vi "相机1初始化.vi"() -> (1 "Session Out":T2, 2 "Image":T1, 3 "相机1状态":bool, 4 "error out":errorcluster)   [LabVIEW 2014]
uses:
  <vilib>/userdefined/High Color/IMAQdx.ctl
  <vilib>/vision/Image Controls.llb/IMAQ Image.ctl
  Controls/MsgAction.ctl
  Global.vi
  <vilib>/vision/driver/NI_Vision_Acquisition_Software.lvlib
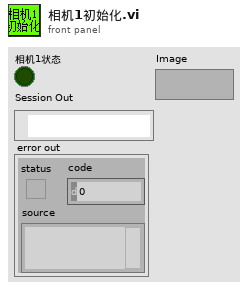
[diagram p1: front panel]
types:
  T1 = typedef "IMAQ Image.ctl" = refnum<image>
  T2 = typedef "IMAQdx.ctl" = refnum<k21>
  T3 = typedef "MsgAction.ctl" = enum16{"初始化", "添加消息", "区分结果添加消息", "清空消息", "获取消息"}
  T4 = typedef "OtherSpec.ctl" = cluster{"其它勾选类规格":T5, "其它数据类规格":T6, "相机名称":T7, "参数":cluster{"Mark1曝光时间":i32, "Mark2曝光时间":i32, "二维码曝光时间":i32}}
  T5 = typedef "其它勾选类规格.ctl" = cluster{"保存图片":bool, "上传设备状态数据":bool, "保存数据":bool, "开机默认开启监控摄像头":bool, "启用mark拍照 ":bool}
  T6 = typedef "其他数据类规格.ctl" = cluster{"相机1像素-毫米换算系数":dbl, "相机2像素-毫米换算系数":dbl, "D盘剩余空间预警(G)":dbl, "视频最长录制时间(秒)":dbl}
  T7 = typedef "相机名称品牌使用状态.ctl" = cluster{"相机1名称":T2, "相机2名称":T2, "Cam1启用":bool, "Cam2启用":bool, "Basler1":bool, "Basler2":bool}
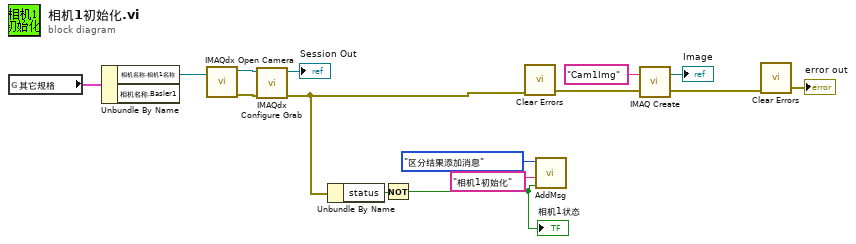
[diagram p0: block diagram]
diagram:
  n1 = global read "Global.vi" "其它规格"() -> (w8:T4)
  n2 = Unbundle By Name(w8) -> ("相机名称.相机1名称"=w9:T2)  [unwired: 1 out]
  n3 = call <vilib>:"IMAQdx Open Camera.vi"("Session In"=w9) -> ("error out"=w14:errorcluster, "Session Out"=w13:T2)  [unwired: 9 in]
  n4 = call <vilib>:"IMAQdx Configure Grab.vi"("error in"=w14, "Session In"=w13) -> ("error out"=w1:errorcluster, "Session Out"=→"Session Out":T2)  [unwired: 8 in]
  n5 = Unbundle By Name(w1) -> ("status"=w10:bool)
  n6 = Not(x=w10) -> (.not. x?=w15:bool)
  "相机1状态" <- w15
  n7 = call <vilib>:"Clear Errors.vi"("error in (no error)"=w1) -> ("error out"=w3:errorcluster)  [unwired: 5 in, 1 out]
  n8 = call "AddMsg.vi"("Result"=w15, "添加消息"="相机1初始化" ("消息显示"), "消息Action"=MsgAction."区分结果添加消息") -> ()  [unwired: 1 in, 1 out]
  n9 = call "IMAQ Create"("Image Name"="Cam1Img", "error in (no error)"=w3) -> ("New Image"=→"Image":T1, "error out"=w6:errorcluster)  [unwired: 3 in]
  n10 = call <vilib>:"Clear Errors.vi"("error in (no error)"=w6) -> ("error out"=→"error out":errorcluster)  [unwired: 5 in, 1 out]
